vi "Send.vi"(7 "Message Priority (Normal)":T1=enum."Normal", 8 "error in (no error)":errorcluster, 9 "Message":refnum<class "Message.lvclass">, 10 "Actor in":refnum<class "Actor.lvclass">, 11 "Instrument Sequencer Sender in":refnum<class "Instrument Sequencer Sender Msg.lvclass">) -> (0 "error out":errorcluster, 1 "Dropped?":bool, 2 "Actor out":refnum<class "Actor.lvclass">)   [LabVIEW 2020, in "Instrument Handler.lvlib" / "Instrument Sequencer Sender Msg.lvclass"]
doc: "Send a Message somewhere through the Publisher. \n\nThis implementation sends a message to a Sequencer Core."
uses:
  Instrument Sequencer Sender Msg.lvclass
  PPL/HDH.Actor Framework.Core.Actor.lvlibp/1abvi3w/vi.lib/ActorFramework/Message Enqueuer/Message Priority.ctl
  PPL/HDH.Actor Framework.Core.Actor.lvlibp/1abvi3w/vi.lib/ActorFramework/Message/Message.lvclass
  PPL/HDH.Actor Framework.Core.Actor.lvlibp/1abvi3w/vi.lib/ActorFramework/Actor/Actor.lvclass
  Instrument Sequencer Sender Msg.lvclass/Instrument Sequencer Sender Msg.ctl
  PPL/HDH.Actor Framework.Core.Sequencer.lvlibp/Sequencer Core/Sequencer Core.lvclass
  PPL/HDH.Actor Framework.Core.Actor.lvlibp/1abvi3w/vi.lib/ActorFramework/Message Enqueuer/Message Enqueuer.lvclass
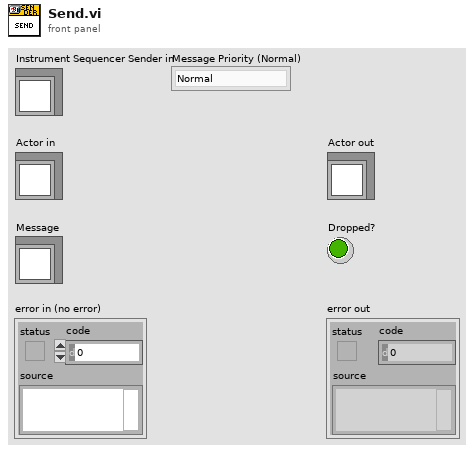
[diagram p1: front panel]
types:
  T1 = typedef "HDH.Actor Framework.Core.Actor.lvlibp/Message Enqueuer.lvclass/Message Priority.ctl" = enum16{"Low", "Normal", "High"}
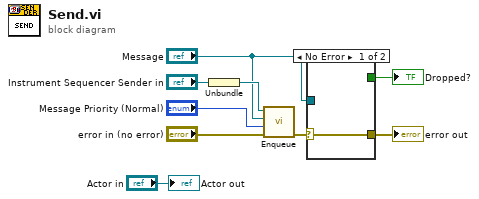
[diagram p0: block diagram]
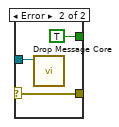
[diagram p2: hidden frame]
diagram:
  n1 = Unbundle("Instrument Sequencer Sender in") -> (w8:refnum<class "Sequencer Core.lvclass">)
  n2 = call "Enqueue.vi"("error in (no error)"="error in (no error)", "Message Priority"="Message Priority (Normal)", "Message"="Message", "Sequencer Core in"=w8) -> ("error out"=w3:errorcluster)  [unwired: 6 in, 1 out]
  n3 = case shown="No Error" w3 {
    selector: w3 -> [w10 w12]
    tunnel: "Message" -> [_ w13]
    tunnel: [w10 w12] -> w2
    tunnel: [_ TRUE] -> w1
    frame No Error {
    }
    frame Error {
      n4 = call-dynamic "Drop Message Core.vi"("Message in"=w13) -> ()  [unwired: 11 in]
    }
  }
  "error out" <- w2
  "Dropped?" <- w1
  "Actor out" <- "Actor in"
